vi "PlugIn AO.vi"(6 "String Value":string, 10 "Channel":T2=enum."Invalid", 11 "Menu":T1=enum."get") -> ()   [LabVIEW 2019]
uses:
  AO Update Ops.ctl
  <vilib>/Rock Robotics/WPI/AnalogOutput/WPI_AnalogOutputChannel.ctl
panel:
  # "Don't place this VI anywhere\nin your API code. It needs to\nbe a dynamically loaded\nwrapper of the main global"
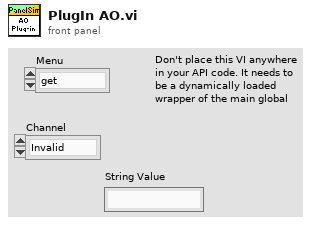
[diagram p1: front panel]
types:
  T1 = typedef "AO Update Ops.ctl" = enum16{"set init", "set value", "JSON update", "set name", "transmit initial", "get", "delete", "reset"}
  T2 = typedef "WPI_AnalogOutputChannel.ctl" = enum8{"AO MXP 0", "AO MXP 1", "Invalid"}
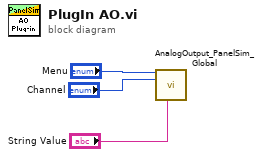
[diagram p0: block diagram]
diagram:
  n1 = call "AnalogOutput_PanelSim_Global.vi"("menu"="Menu", "AO Channel"="Channel", "JSON"="String Value") -> ()  [unwired: 11 in, 2 out]
